vi "Write VISA resource name.vi"(8 "error in (no error)":errorcluster, 10 "VISA resource name":refnum<visa-resource-name>, 11 "Abstract Camera in":refnum<class "Abstract Camera.lvclass">) -> (0 "error out":errorcluster, 3 "Abstract Camera out":refnum<class "Abstract Camera.lvclass">)   [LabVIEW 2019, in "Abstract Camera.lvclass"]
uses:
  Abstract Camera.lvclass
  Abstract Camera.lvclass/Abstract Camera.ctl
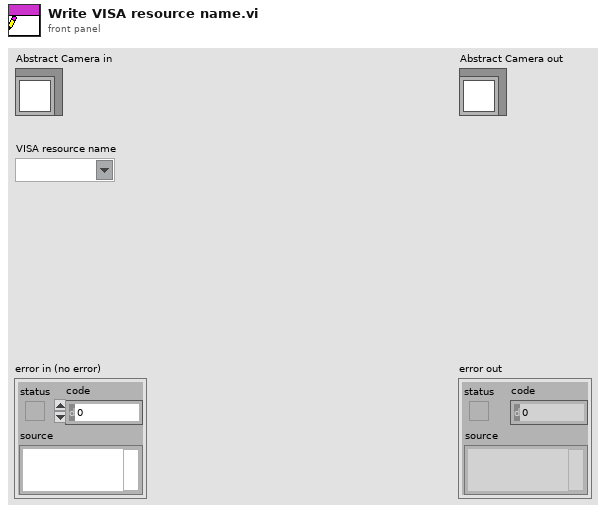
[diagram p1: front panel]
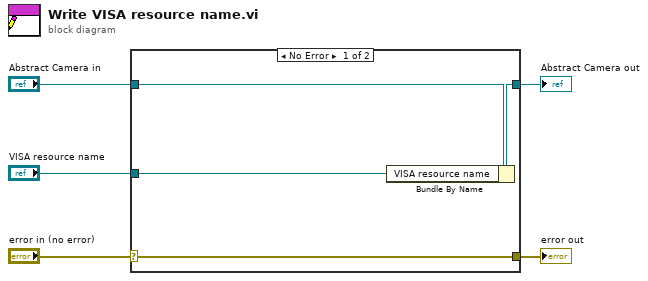
[diagram p0: block diagram]
diagram:
  n1 = case shown="No Error" "error in (no error)" {
    selector: "error in (no error)" -> [w9 w10]
    tunnel: [w9 w10] -> w4
    tunnel: [w7 w11] -> w2
    tunnel: "Abstract Camera in" -> [w8 w11]
    tunnel: "VISA resource name" -> [w6 _]
    frame No Error {
      n2 = Bundle By Name(cluster=w8, "VISA resource name"=w6) -> (w7:refnum<class "Abstract Camera.lvclass">)
    }
    frame Error {
    }
  }
  "error out" <- w4
  "Abstract Camera out" <- w2
